vi "test_libssh2_agent_get_identity.vi"() -> ()   [LabVIEW 2013, in "libssh2_integration_tests.lvlib"]
uses:
  libssh2_integration_tests.lvlib
  libssh2/libssh2_init_default.vi
  <vilib>/addons/_JKI Toolkits/Caraya/classes/Assert/Assert Equal Value_Variant.vi
  <vilib>/addons/_JKI Toolkits/Caraya/classes/Test/Test.lvclass
  <vilib>/addons/_JKI Toolkits/Caraya/classes/Assert/Assert.lvclass
  Agent Fixture/Agent Fixture.lvclass
  libssh2/libssh2.lvlib
panel:
  out "error out":errorcluster
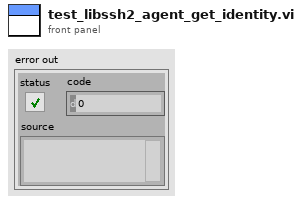
[diagram p1: front panel]
types:
  T1 = typedef "libssh2.lvlib/Session Refnum.ctl" = refnum<k1>
  T2 = typedef "libssh2.lvlib/Agent Refnum.ctl" = refnum<k1>
  T3 = typedef "libssh2.lvlib/Agent Public Key Refnum.ctl" = refnum<k1>
  T4 = typedef "libssh2.lvlib/libssh2_agent_publickey.ctl" = cluster{"magic":u32, "node":u64, "blob":u8[], "blob_len":u64, "comment":string}
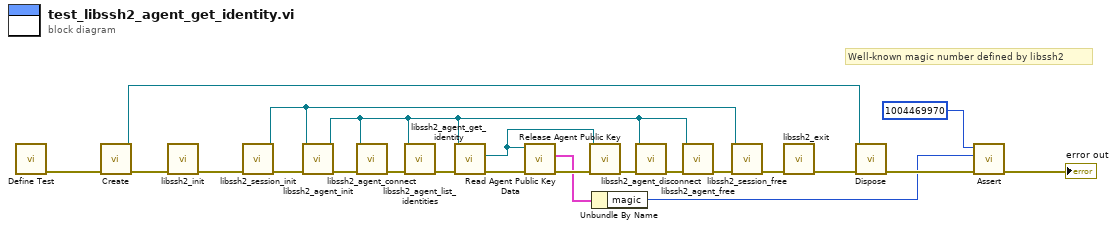
[diagram p0: block diagram]
diagram:
  # "Well-known magic number defined by libssh2"
  n1 = call <vilib>:"Define Test.vi"() -> ("error out"=w23:errorcluster)  [unwired: 10 in, 1 out]
  n2 = call "Create.vi"("error in (no error)"=w23) -> ("error out"=w22:errorcluster, "Agent Fixture"=w3:refnum<class "Agent Fixture.lvclass">)  [unwired: 9 in]
  n3 = call-poly "libssh2_init.vi"("error in (no error)"=w22) -> ("error out"=w20:errorcluster)  [unwired: 10 in]
  n4 = call "libssh2_session_init.vi"("error in (no error)"=w20) -> ("error out"=w18:errorcluster, "session"=w15:T1)  [unwired: 9 in]
  n5 = call "libssh2_agent_init.vi"("error in (no error)"=w18, "session"=w15) -> ("error out"=w16:errorcluster, "agent"=w4:T2)  [unwired: 8 in]
  n6 = call "libssh2_agent_connect.vi"("error in (no error)"=w16, "agent"=w4) -> ("error out"=w6:errorcluster)  [unwired: 9 in]
  n7 = call "libssh2_agent_list_identities.vi"("error in (no error)"=w6, "agent"=w4) -> ("error out"=w13:errorcluster)  [unwired: 9 in]
  n8 = call "libssh2_agent_get_identity.vi"("error in (no error)"=w13, "agent"=w4) -> ("error out"=w12:errorcluster, "store"=w9:T3)  [unwired: 7 in, 1 out]
  n9 = call "Read Agent Public Key Data.vi"("error in (no error)"=w12, "agent public key"=w9) -> ("error out"=w11:errorcluster, "value"=w8:T4)  [unwired: 8 in]
  n10 = call "Release Agent Public Key.vi"("error in (no error)"=w11, "agent public key"=w9) -> ("error out"=w10:errorcluster)  [unwired: 9 in]
  n11 = Unbundle By Name(w8) -> ("magic"=w2:u32)
  n12 = call "libssh2_agent_disconnect.vi"("error in (no error)"=w10, "agent"=w4) -> ("error out"=w5:errorcluster)  [unwired: 9 in]
  n13 = call "libssh2_agent_free.vi"("error in (no error)"=w5, "agent"=w4) -> ("error out"=w14:errorcluster)  [unwired: 9 in]
  n14 = call "libssh2_session_free.vi"("error in (no error)"=w14, "session"=w15) -> ("error out"=w17:errorcluster)  [unwired: 9 in]
  n15 = call "libssh2_exit.vi"("error in (no error)"=w17) -> ("error out"=w19:errorcluster)  [unwired: 10 in]
  n16 = call "Dispose.vi"("error in (no error)"=w19, "Agent Fixture in"=w3) -> ("error out"=w21:errorcluster)  [unwired: 9 in]
  n17 = call-poly <vilib>:"Assert.vi"("error in (no error)"=w21, "Y"=w2, "X"=u32 1004469970) -> ("error out"=→"error out":errorcluster)  [unwired: 7 in, 1 out]
